vi "Configure_Target.vi"(6 "Mode":T1, 8 "error in":errorcluster, 9 "Destination":string, 10 "Target":string, 11 "MLTFNC in":refnum<class "MLTFNC.lvclass">) -> (0 "error out":errorcluster, 3 "MLTFNC out":refnum<class "MLTFNC.lvclass">)   [LabVIEW 2019, in "MLTFNC.lvlib" / "MLTFNC.lvclass"]
uses:
  Library/MLTFNC.lvclass
  C:/Users/Public/Documents/Development/builds/Instruments/Instruments.lvlibp/Library/Instruments.lvclass
  Custom Controls/Mode.ctl
  Library/MLTFNC.lvclass/MLTFNC.ctl
  builds/Instruments/Instruments.lvlibp/Private/Polymorphic/Special/Event from String.vi
  builds/Instruments/Instruments.lvlibp/Accessors/Command with Logging.vi
  builds/Instruments/Instruments.lvlibp/Library/Instruments.lvclass
  builds/Instruments/Instruments.lvlibp
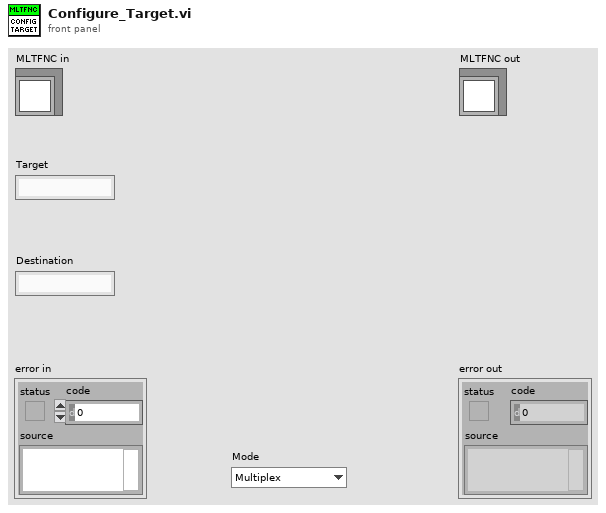
[diagram p1: front panel]
types:
  T1 = typedef "MLTFNC.lvlib/MLTFNC.lvclass/Mode.ctl" = enum16{"Multiplex"}
  T2 = cluster{"Timestamp":timestamp, "Description":string, "Data":string}
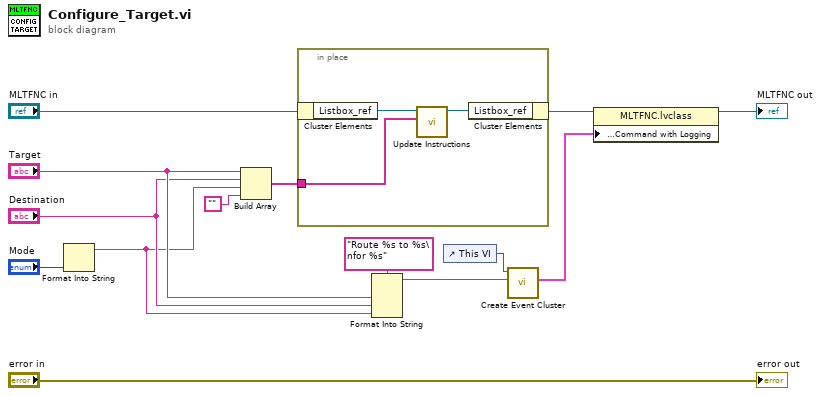
[diagram p0: block diagram]
diagram:
  n1 = Format Into String("Mode") -> (resulting string=w1:string)  [unwired: 3 in, 1 out]
  n2 = Build Array("Target", "Destination", w1, "") -> (w9:string[])
  n3 = in-place {
    in-place-border: w9 -> [w15]
    n4 = in-place-cluster #1("MLTFNC in") -> ("Listbox_ref"=w17:refnum<vi>)
    n5 = call "Update Instructions.vi"("Instructions"=w15, "referencein"=w17) -> ("reference out"=w16:refnum<vi>)  [unwired: 9 in]
    n6 = in-place-cluster #1("Listbox_ref"=w16) -> (w10:refnum<class "MLTFNC.lvclass">)
  }
  n7 = Format Into String(format string="Route %s to %s\nfor %s", "Target", "Destination", w1) -> (resulting string=w6:string)  [unwired: 2 in, 1 out]
  n8 = control-ref of="This VI"() -> (w4:refnum<vi>)
  n9 = call-poly "Create Event Cluster.vi"("Value"=w6, "VI Refnum"=w4) -> ("Event Data"=w5:T2)  [unwired: 9 in]
  n10 = property class="MLTFNC.lvclass"(reference=w10, "Accessors:Logging:Command with Logging"=w5) -> (reference out=→"MLTFNC out":refnum<class "MLTFNC.lvclass">)  [unwired: 1 in, 1 out]
  "error out" <- "error in"
